vi "ui_main.vi"() -> ()   [LabVIEW 2015]
uses:
  type_definitions/ui_data.ctl
  globals/global_all_ui_loop_stop.vi
  support_vis/user_event_stop/user_event_stop.lvlib
  support_vis/message_queue/message_queue.lvlib
panel:
  in  "Connect to RT":bool caption="连接实时终端"
  out "Connected?":bool caption="已连接？"
  in  "Controller Address":string="192.168.17.102" caption="控制器地址"
  in  "Device Tree":string[](tree)=["FCXF-X-03-S05"] caption="设备列表"
  in  "Settings Tab":enum32{"实时数据", "System Monitoring"}(tab) caption="设置选项卡"
  out "Live Data":waveform(dbl)[](graph) caption="实时数据"
  out "Number of Data Files":u32 caption="数据文件数："
  out "Scan Engine Period (ms)":u32 caption="扫描引擎周期（ms）："
  out "Free Memory(Mb)":dbl(graph) caption="剩余内存（Mb）"
  out "System Time":timestamp caption="系统时间" format="%<%Y/%m/%d %H:%M:%S>T"
  out "Resource Utilization (%)":T1(graph) caption="资源利用率(%)"
  out "Controller Operating Status":string="控制器工作状态" caption="控制器运行状态"
  out "Error Infomation":string="错误信息" caption="错误信息"
  in  "Exit":bool caption="退出"
  # "中小跨径桥梁健康监测系统实时数据预览"
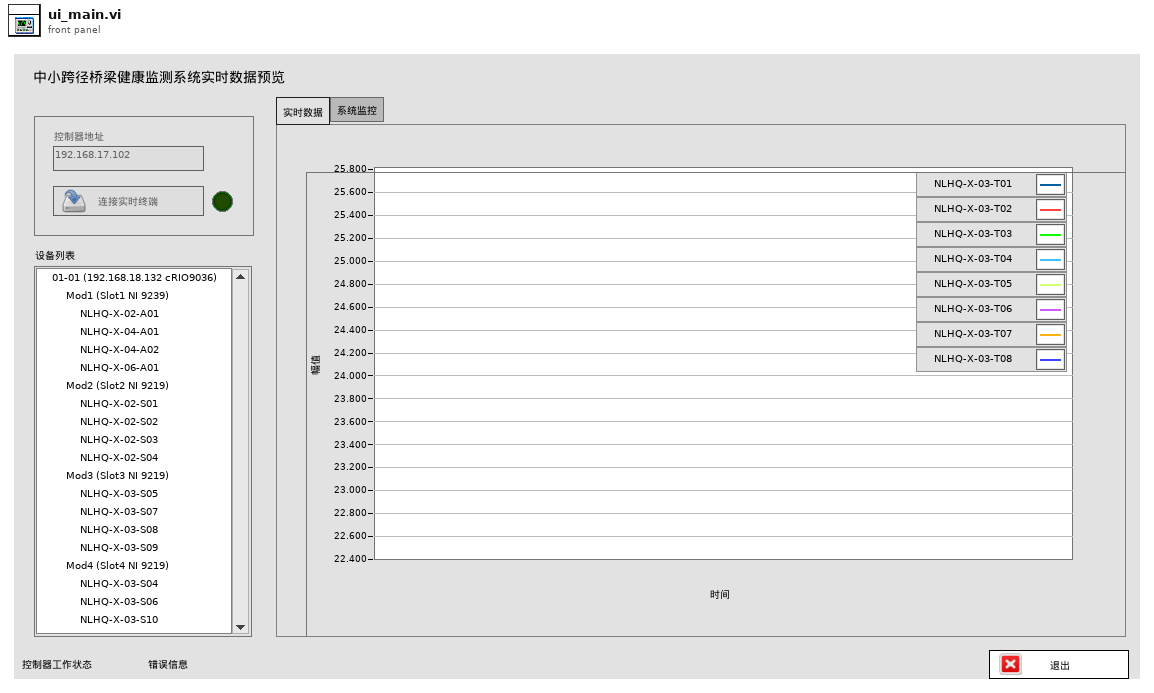
[diagram p1: front panel]
types:
  T1 = cluster{"CPU #1 Usage":dbl, "CPU #2 Usage":dbl, "Driver Space":dbl}
  T2 = typedef "ui_data.ctl" = cluster{"Connected? Ref":refnum<vi>, "Controller Address Ref":refnum<vi>, "Error Infomation Ref":refnum<vi>, "Scan Engine Period (ms) Ref":refnum<vi>, "Number of Data Files Ref":refnum<vi>, "System Time Ref":refnum<vi>, "Free Memory Ref":refnum<vi>, "Device Tree Ref":refnum<vi>, "Controller Working Status Ref":refnum<vi>, "Connect to RT":refnum<vi>, "Exit":refnum<vi>, "Tab Ref":refnum<vi>, "Live Data Ref":refnum<vi>, "Resource Utilization (%) Ref":refnum<vi>}
  T3 = typedef "All Host Message Queues.ctl" = cluster{"UI":refnum<queue>}
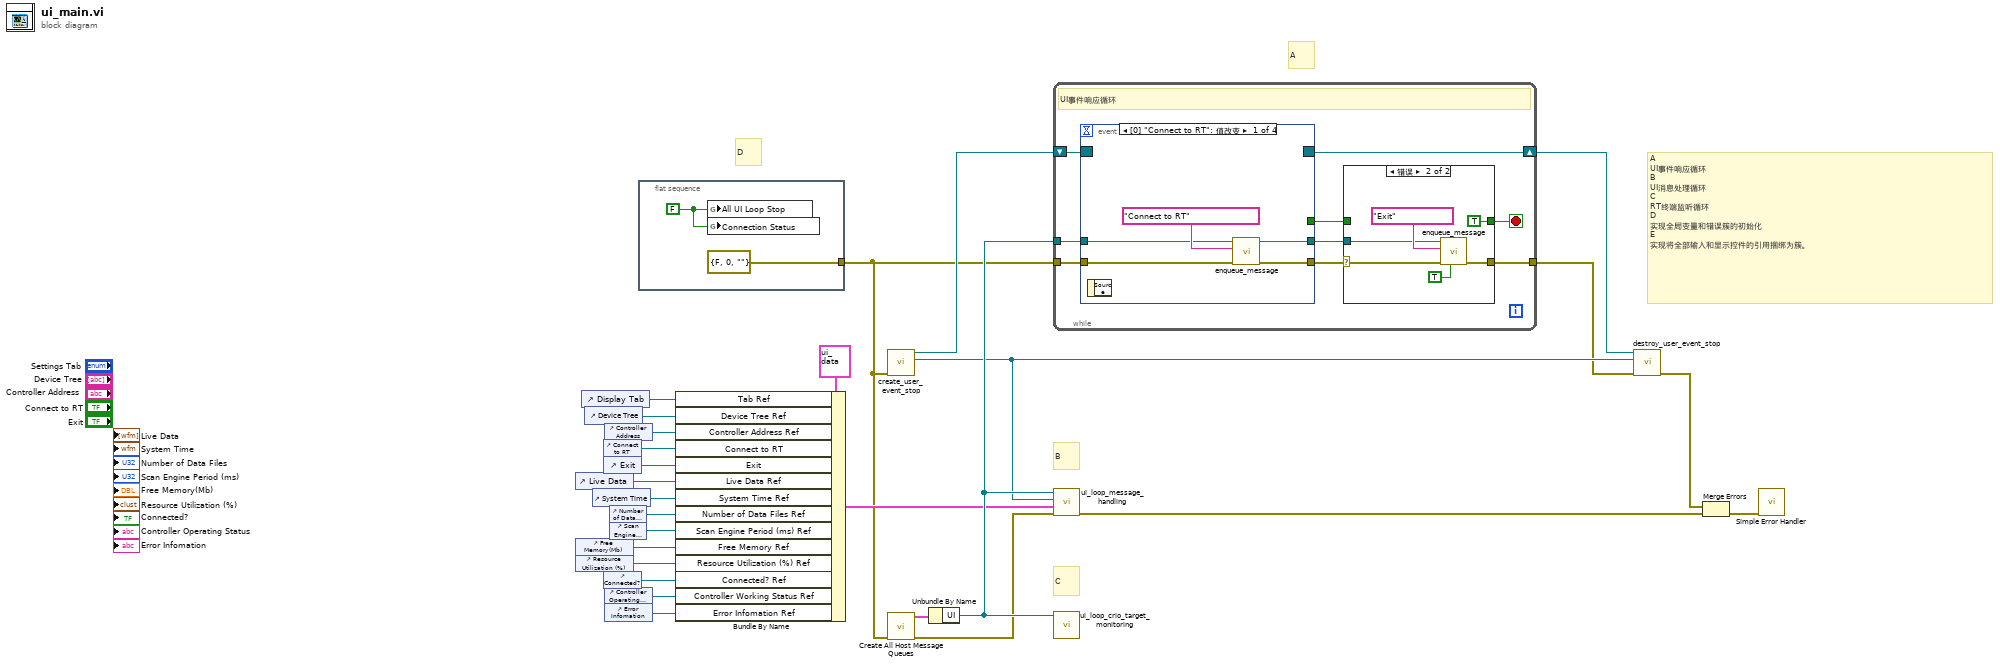
[diagram p0: block diagram]
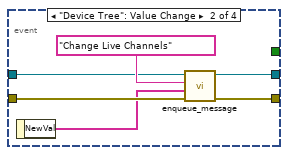
[diagram p3: hidden frame]
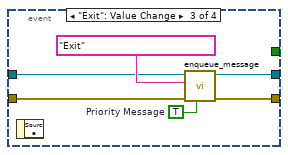
[diagram p4: hidden frame]
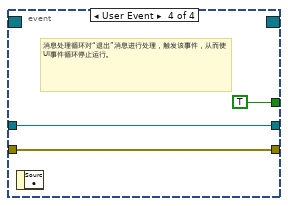
[diagram p5: hidden frame]
diagram:
  # "C"
  # "A"
  # "B"
  # "D"
  # "A\nUI事件响应循环\nB\nUI消息处理循环\nC\nRT终端监听循环\nD\n实现全局变量和错误簇的初始化\nE\n实现将全部输入和显示控件的引用捆绑为簇。"
  n1 = control-ref of="Live Data"() -> (w14:refnum<vi>)
  n2 = control-ref of="Free Memory(Mb)"() -> (w10:refnum<vi>)
  n3 = control-ref of="Resource Utilization (%)"() -> (w9:refnum<vi>)
  n4 = control-ref of="Display Tab"() -> (w2:refnum<vi>)
  n5 = control-ref of="Device Tree"() -> (w1:refnum<vi>)
  n6 = control-ref of="System Time"() -> (w13:refnum<vi>)
  n7 = control-ref of="Connect to RT"() -> (w5:refnum<vi>)
  n8 = control-ref of="Exit"() -> (w3:refnum<vi>)
  n9 = control-ref of="Connected?"() -> (w8:refnum<vi>)
  n10 = control-ref of="Controller Address"() -> (w4:refnum<vi>)
  n11 = control-ref of="Controller Operating Status"() -> (w7:refnum<vi>)
  n12 = control-ref of="Error Infomation"() -> (w6:refnum<vi>)
  n13 = control-ref of="Number of Data Files"() -> (w12:refnum<vi>)
  n14 = control-ref of="Scan Engine Period (ms)"() -> (w11:refnum<vi>)
  n15 = flat-sequence {
    tunnel: [errorcluster {"status"=FALSE, "code"=0, "source"=""} ("error in (no error)")] -> w16
    frame #0 {
      w28 = FALSE
      n16 = global write "global_all_ui_loop_stop.vi" "All UI Loop Stop"(w28) -> ()
      n17 = global write "global_all_ui_loop_stop.vi" "Connection Status"(w28) -> ()
    }
  }
  n18 = Bundle By Name(cluster=T2 {"Connected? Ref"=refnum, "Controller Address Ref"=refnum, "Error Infomation Ref"=refnum, "Scan Engine Period (ms) Ref"=refnum, "Number of Data Files Ref"=refnum, "System Time Ref"=refnum, "Free Memory Ref"=refnum, "Device Tree Ref"=refnum, "Controller Working Status Ref"=refnum, "Connect to RT"=refnum, "Exit"=refnum, "Tab Ref"=refnum, "Live Data Ref"=refnum, "Resource Utilization (%) Ref"=refnum} ("Measurement UI Controls"), "Tab Ref"=w2, "Device Tree Ref"=w1, "Controller Address Ref"=w4, "Connect to RT"=w5, "Exit"=w3, "Live Data Ref"=w14, "System Time Ref"=w13, "Number of Data Files Ref"=w12, "Scan Engine Period (ms) Ref"=w11, "Free Memory Ref"=w10, "Resource Utilization (%) Ref"=w9, "Connected? Ref"=w8, "Controller Working Status Ref"=w7, "Error Infomation Ref"=w6) -> (w17:T2)
  n19 = call "create_user_event_stop.vi"("error in (no error)"=w16) -> ("User Event - Stop"=w20:refnum<user-event>, "Stop Event Registration Refnum"=w27:refnum<event-registration>)  [unwired: 8 in, 1 out]
  n20 = call "Create All Host Message Queues.vi"("error in (no error)"=w16) -> ("error out"=w24:errorcluster, "Message Queues out"=w26:T3)  [unwired: 9 in]
  n21 = Unbundle By Name(w26) -> ("UI"=w25:refnum<queue>)
  n22 = while {
    tunnel: w25 -> [w34]
    shift-right: [w33] -> w18
    shift-left: w27 -> [w35]
    tunnel: w16 -> [w32]
    tunnel: [w30] -> w15
    stop <- w37 stop-if-true
    # "UI事件响应循环"
    n23 = event shown="[0] \"Connect to RT\": 值改变" {
      selector: w35 -> [_ _ _ _]
      dyn-events: [_ _ _ _] -> w33
      timeout: _ -> [_ _ _ _]
      tunnel: [_ _ _ TRUE ("Discard?")] -> w38
      tunnel: w34 -> [w49 w56 w60 w64]
      tunnel: [w51 w53 w63 w65] -> w36
      tunnel: w32 -> [w48 w55 w59 w65]
      tunnel: [w47 w54 w58 w64] -> w31
      event "Connect to RT": Value Change {
        n24 = event-data() -> ()  [unwired: 1 in, 1 out]
        n25 = call "enqueue_message.vi"("error in (no error)"=w48, "Message"="Connect to RT", "Message Queue"=w49) -> ("error out"=w51:errorcluster, "dup Message Queue"=w47:refnum<queue>)  [unwired: 7 in]
      }
      event "Device Tree": Value Change {
        n26 = event-data() -> ("NewVal"=w52:string[])  [unwired: 1 in]
        n27 = call "enqueue_message.vi"("error in (no error)"=w55, "Message Data"=w52, "Message"="Change Live Channels", "Message Queue"=w56) -> ("error out"=w53:errorcluster, "dup Message Queue"=w54:refnum<queue>)  [unwired: 6 in]
      }
      event "Exit": Value Change {
        w61 = TRUE  # Priority Message
        n28 = event-data() -> ()  [unwired: 1 in, 1 out]
        n29 = call "enqueue_message.vi"("Priority Message? (F)"=w61, "error in (no error)"=w59, "Message"="Exit", "Message Queue"=w60) -> ("error out"=w63:errorcluster, "dup Message Queue"=w58:refnum<queue>)  [unwired: 6 in]
      }
      event User Event {
        # "消息处理循环对“退出”消息进行处理，触发该事件，从而使UI事件循环停止运行。"
        n30 = event-data() -> ()  [unwired: 1 in, 1 out]
      }
    }
    n31 = case shown="错误" w36 {
      selector: w36 -> [w39 w42]
      tunnel: [w40 TRUE ("Discard?")] -> w37
      tunnel: w38 -> [w40 _]
      tunnel: w31 -> [_ w43]
      tunnel: [w39 w41] -> w30
      frame No Error {
        # "无错误"
      }
      frame Error {
        # "出现错误时，发送“退出”消息，使循环停止运行。"
        n32 = call "enqueue_message.vi"("Priority Message? (F)"=TRUE ("Discard?"), "error in (no error)"=w42, "Message"="Exit", "Message Queue"=w43) -> ("error out"=w41:errorcluster)  [unwired: 6 in, 1 out]
      }
    }
  }
  n33 = call "ui_loop_message_handling.vi"("error in (no error)"=w24, "UI Control Refs Cluster"=w17, "User Event - Stop"=w20, "UI Message Queue Ref"=w25) -> ("error out"=w23:errorcluster)  [unwired: 7 in]
  n34 = call "ui_loop_crio_target_monitoring.vi"("Message Queue Reference"=w25) -> ()  [unwired: 11 in]
  n35 = call "destroy_user_event_stop.vi"("Stop Event Registeration"=w18, "User Event - Stop"=w20, "error in (no error)"=w15) -> ("error out"=w19:errorcluster)  [unwired: 7 in]
  n36 = Merge Errors(w19, w23) -> (w21:errorcluster)
  n37 = call <vilib>:"Simple Error Handler.vi"("error in (no error)"=w21) -> ()  [unwired: 4 in, 5 out]
